vi "ULx Create 1D Digital port Waveform (NSamp).vi"(0 "t0":ext format="%#_10g", 5 "dt":dbl, 7 "data Array":dbl[][](array[numeric]) format="%0.2f", 9 "port widths":i32[](array[numeric]), 11 "error in":errorcluster) -> (4 "data":digitalwaveform[](array[waveform]), 15 "error out":errorcluster)   [LabVIEW 2020]
uses:
  DWDT Analog to Digital.vi
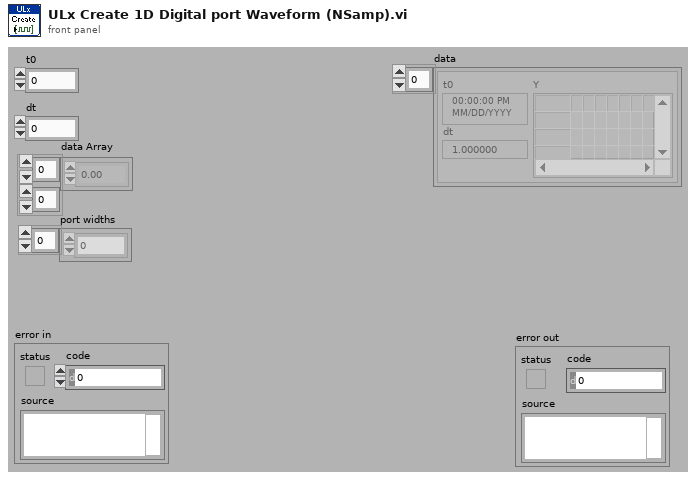
[diagram p1: front panel]
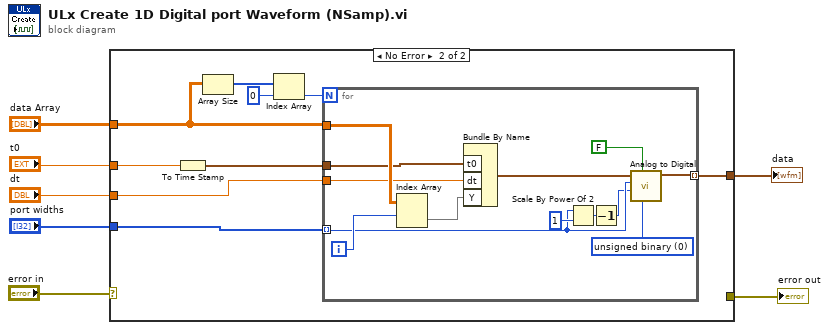
[diagram p0: block diagram]
diagram:
  n1 = case shown="No Error" "error in" {
    selector: "error in" -> [w8 _]
    tunnel: [w8 _] -> w6
    tunnel: "data Array" -> [_ w13]
    tunnel: "t0" -> [_ w12]
    tunnel: "dt" -> [_ w11]
    tunnel: [_ w10] -> w2
    tunnel: "port widths" -> [_ w9]
    frame Error {
    }
    frame No Error {
      n2 = To Time Stamp(1:w12) -> (0:w17:timestamp)
      n3 = Array Size(array=w13) -> (size(s)=w14:i32[])
      n4 = Index Array(array=w14, index=0) -> (element=w16:i32)
      n5 = for {
        N: w16 -> [_]
        tunnel: w13 -> [w30]
        tunnel: [w25] -> w10 mode=indexing
        tunnel: w17 -> [w28]
        tunnel: w11 -> [w27]
        tunnel: w9 -> [w21] mode=indexing
        i -> [w26]
        w23 = u16 0 items=["unsigned binary", "offset binary", "2's complement"] ("data format (offset binary)")
        n6 = Index Array(array=w30, index (row)=w26) -> (element=w29:dbl[])  [unwired: 1 in]
        n7 = Bundle By Name("t0"=w28, "dt"=w27, "Y"=w29) -> (w18:waveform(dbl))  [unwired: 1 in]
        n8 = Scale By Power Of 2(n=w21, x=u32 1) -> (x*2^n=w20:u32)
        n9 = Decrement(x=w20) -> (x-1=w19:u32)
        n10 = call-poly "Analog to Digital.vi"("data format (offset binary)"=w23, "compress digital (T)"=FALSE, "full-scale range (pk-pk)"=w19, "resolution (16 bit)"=w21, "analog waveform"=w18) -> ("digital waveform"=w25:digitalwaveform)  [unwired: 3 in, 3 out]
      }
    }
  }
  "error out" <- w6
  "data" <- w2
